vi "Arduino_control_GCFS.vi"(2 "error in (no error)":errorcluster, 3 "Arguments":string, 4 "Connection":bool, 5 "Port":refnum<visa-resource-name>) -> (0 "error out":errorcluster, 1 "Connection":bool)   [LabVIEW 2024]
uses:
  5242033b-70ca-4bd5-889b-60dceb38dbd2.vi
  <vilib>/regexp/Match Regular Expression.xnode
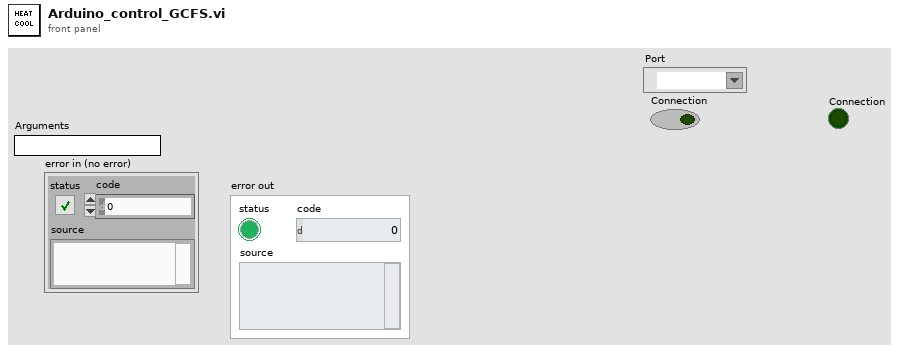
[diagram p1: front panel]
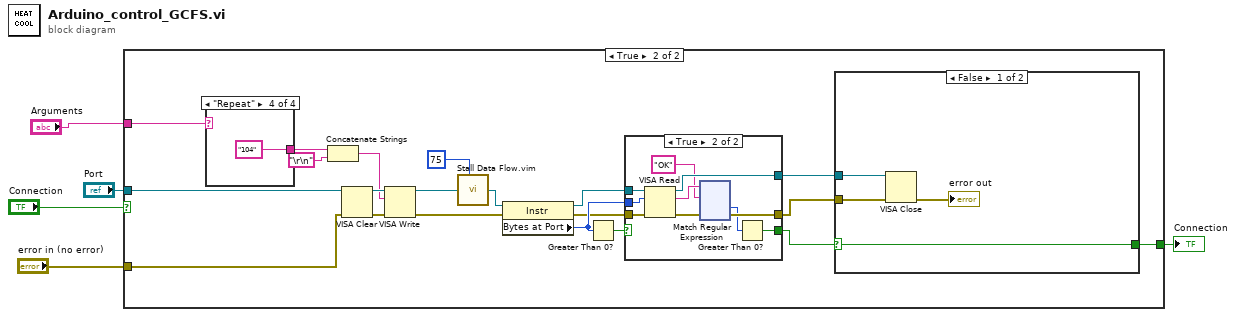
[diagram p0: block diagram]
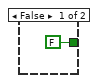
[diagram p2: hidden frame]
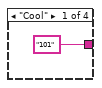
[diagram p3: hidden frame]
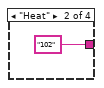
[diagram p4: hidden frame]
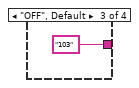
[diagram p5: hidden frame]
diagram:
  n1 = case shown="True" "Connection" {
    tunnel: "Port" -> [_ w23]
    tunnel: [FALSE w9] -> w3
    tunnel: "Arguments" -> [_ w7]
    tunnel: "error in (no error)" -> [_ w8]
    frame False {
    }
    frame True {
      n2 = case shown="\"Repeat\"" w7 {
        tunnel: ["101" ("string") "102" ("string") "103" ("string") "104" ("string")] -> w14
        frame "Cool" {
        }
        frame "Heat" {
        }
        frame "OFF", Default {
        }
        frame "Repeat" {
        }
      }
      n3 = Concatenate Strings(w14, "\r\n") -> (w12:string)
      n4 = VISA Clear(VISA resource name=w23, error in (no error)=w8) -> (VISA resource name out=w25:refnum<visa-resource-name>, error out=w24:errorcluster)
      n5 = VISA Write(VISA resource name=w25, write buffer=w12, error in (no error)=w24) -> (VISA resource name out=w21:refnum<visa-resource-name>, error out=w19:errorcluster)  [unwired: 1 out]
      n6 = call "Stall Data Flow.vim"("value in"=w21, "milliseconds to wait"=u32 75) -> ("value out"=w20:refnum<visa-resource-name>)  [unwired: 1 out]
      n7 = property class="Instr"(reference=w20, error in=w19) -> (reference out=w18:refnum<visa-resource-name>, error out=w16:errorcluster, "Bytes at Port"=w17:u32)
      n8 = Greater Than 0?(x=w17) -> (x > 0?=w26:bool)
      n9 = case shown="True" w26 {
        selector: w26 -> [w36 _]
        tunnel: w17 -> [_ w48]
        tunnel: w16 -> [w37 w47]
        tunnel: [w38 w46] -> w15
        tunnel: [w37 w41] -> w10
        tunnel: w18 -> [w38 w45]
        tunnel: [w36 w39] -> w11
        frame False {
        }
        frame True {
          n10 = VISA Read(VISA resource name=w45, byte count=w48, error in (no error)=w47) -> (VISA resource name out=w46:refnum<visa-resource-name>, read buffer=w44:string, error out=w43:errorcluster)  [unwired: 1 out]
          n11 = xnode "Match Regular Expression"("input string"=w44, "regular expression"="OK", "error in"=w43) -> ("offset past match"=w40:i32, "error out"=w41:errorcluster)  [unwired: 3 in, 3 out]
          n12 = Greater Than 0?(x=w40) -> (x > 0?=w39:bool)
        }
      }
      n13 = case shown="False" w11 {
        selector: w11 -> [w31 w35]
        tunnel: w15 -> [w34 _]
        tunnel: w10 -> [w32 _]
        tunnel: [w31 w35] -> w9
        frame False {
          n14 = VISA Close(VISA resource name=w34, error in (no error)=w32) -> (error out=→"error out":errorcluster)
        }
        frame True {
        }
      }
    }
  }
  "Connection" <- w3
